vi "Main.vi"(11 "Module Admin":refnum<class "Delacor_lib_QMH_Module Admin.lvclass">) -> ()   [LabVIEW 2018, in "Application.lvlib"]
doc: "This template is based off of the Queued Message Handler design pattern and the Queued Message Handler project template that ships with LabVIEW.\n\nThe main difference is that the queue is private to this module and communication between modules is performed via Broadcast and Request events.\n\nRequest events are wrapped in public API methods and are handled in the Event Handling Loop (EHL) of this VI. Any module can register for Broadcast events sent by this module. The EHL generates messages based on user interface actions.\n\nThe Message Handling Loop (MHL) processes messages generated by the EHL, or by other messages. The messages are string values, so new messages can be added easily to the Message Cases case structure in the MHL. Each message cluster can also provide an optional value for Message Data, which is a variant that can be converted to whatever message-specific data is required.\n_____\nBased on DQMH Project Template 6.1.0.94."
uses:
  Application.lvlib
  <vilib>/Delacor/Delacor QMH/Libraries/Module Admin_class/Delacor_lib_QMH_Module Admin.lvclass
  Module Data--cluster.ctl
  <vilib>/Delacor/Delacor QMH/Libraries/Message Queue_class/Delacor_lib_QMH_Message Queue.lvclass/Delacor_lib_QMH_Message Queue.ctl
  Stop Argument--cluster.ctl
  <vilib>/Delacor/Delacor QMH/Libraries/Module Admin_class/Delacor_lib_QMH_Module Admin.lvclass/Delacor_lib_QMH_Module Admin.ctl
  <vilib>/Delacor/Delacor QMH/Libraries/Message Queue_class/Delacor_lib_QMH_Enqueue Message (Single).vi
  <vilib>/Delacor/Delacor QMH/Libraries/Module Admin_class/Delacor_lib_QMH_Get External Launch.vi
  <vilib>/Delacor/Delacor QMH/Libraries/Message Queue_class/Delacor_lib_QMH_Enqueue Message (Array).vi
  <vilib>/Utility/error.llb/Error Cluster From Error Code.vi
  <vilib>/ErrorRing/Error Ring.xnode
  <vilib>/Delacor/Delacor QMH/Libraries/Message Queue_class/Delacor_lib_QMH_Message Queue.lvclass
  Storage/Storage.lvlib
  DAQ/DAQ.lvlib
panel:
  in  "Virtual keyboard":bool
  out "设备状态":bool
  in  "Export Graph 3":bool
  in  "Export Graph 2":bool
  in  "通讯配置":bool
  in  "Clear Graph":bool
  in  "是否打开串口":bool
  in  "设备通讯":bool
  out "error out":errorcluster
  out "Status":string
  in  "Simulate MHL Error":bool
  in  "Simulate EHL Error":bool
  in  "Ring曲线选择":u16(ring) caption="选择查看曲线" items=["CH01", "CH02", "CH03", "CH04", "CH05", "CH06", "CH07", "CH08"]
  out "最高温度":dbl format="%#.0f℃"
  out "温度监控":T1 {"CH 8" format="%#0.1f℃"; "CH 7" format="%#0.1f℃"; "CH 6" format="%#0.1f℃"; "CH 5" format="%#0.1f℃"; "CH 4" format="%#0.1f℃"; "CH 3" format="%#0.1f℃"; "CH 2" format="%#0.1f℃"; "CH" format="%#0.1f℃"}
  out "Value":dbl caption="Y Value" format="%0.2f"
  out "XYGraph":cluster{"时间":dbl[], "曲线":dbl[]}(graph) caption="-- 温度曲线"
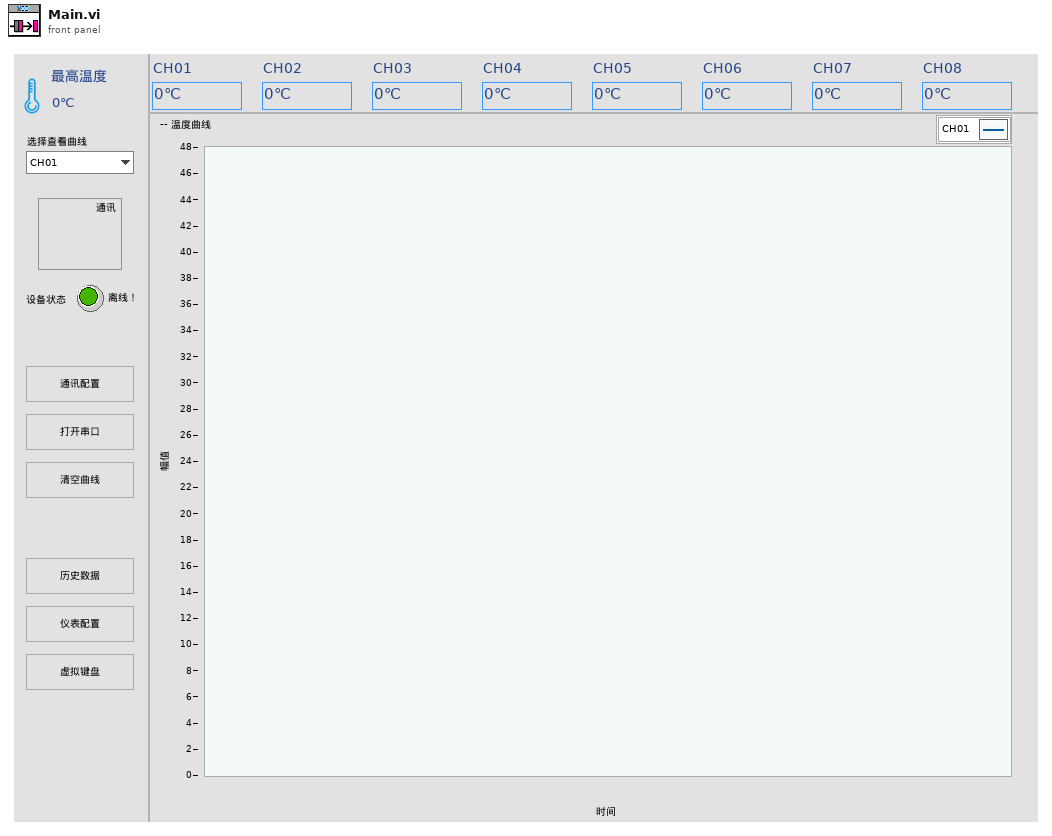
[diagram p1: front panel]
types:
  T1 = cluster{"CH":dbl, "CH 2":dbl, "CH 3":dbl, "CH 4":dbl, "CH 5":dbl, "CH 6":dbl, "CH 7":dbl, "CH 8":dbl}
  T2 = typedef "Storage.lvlib/Broadcast Events--cluster.ctl" = cluster{"Module Did Init":refnum<user-event>, "Status Updated":refnum<user-event>, "Error Reported":refnum<user-event>, "Module Did Stop":refnum<user-event>, "Update Module Execution Status":refnum<user-event>}
  T3 = typedef "DAQ.lvlib/Broadcast Events--cluster.ctl" = cluster{"Module Did Init":refnum<user-event>, "Status Updated":refnum<user-event>, "Error Reported":refnum<user-event>, "Module Did Stop":refnum<user-event>, "Update Module Execution Status":refnum<user-event>}
  T4 = typedef "Application.lvlib/Request Events--cluster.ctl" = cluster{"Stop Module":refnum<user-event>, "Show Panel":refnum<user-event>, "Hide Panel":refnum<user-event>, "Get Module Execution Status":refnum<user-event>, "Show Diagram":refnum<user-event>, "Wakeup or Sleep HL":refnum<user-event>}
  T5 = typedef "Application.lvlib/Module Data--cluster.ctl" = cluster{"Status":string, "TDMS":refnum<k34>}
  T6 = enum32{"invalid lock state", "Not Locked", "Locked (No Password)", "Password-protected"}
  T7 = typedef "Application.lvlib/Stop Argument--cluster.ctl" = cluster{"Origin":string, "Exit via Stop Module Req?":bool, "Wait for Module to stop?":bool}
  T8 = enum32{"Invalid", "Standard", "Closed", "Hidden", "Minimized", "Maximized"}
  T9 = typedef "LVPoint32TypeDef.ctl" = cluster{"Horizontal":i32, "Vertical":i32}
  T10 = cluster{"温度[0]":dbl, "温度[1]":dbl, "温度[2]":dbl, "温度[3]":dbl, "温度[4]":dbl, "温度[5]":dbl, "温度[6]":dbl, "温度[7]":dbl}
  T11 = typedef "LVPositionTypeDef.ctl" = cluster{"Left":i32, "Top":i32}
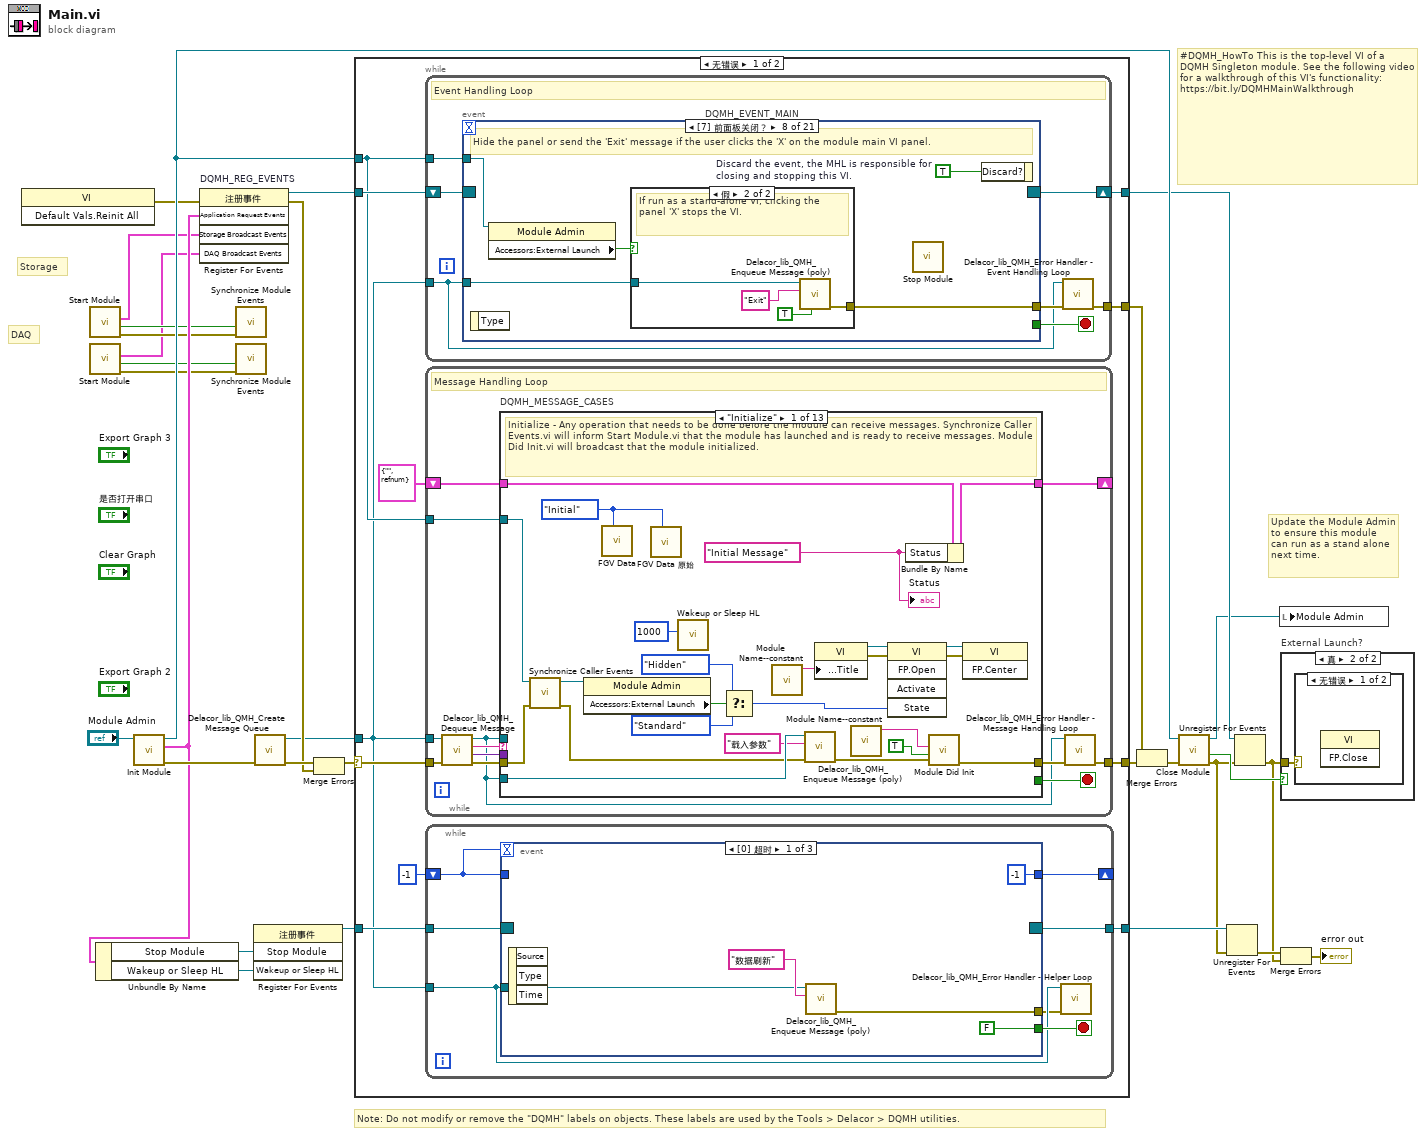
[diagram p0: block diagram]
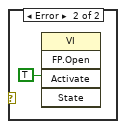
[diagram p3: hidden frame]
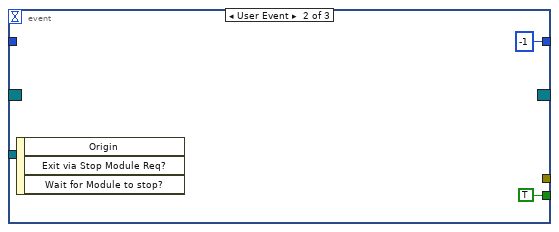
[diagram p4: hidden frame]
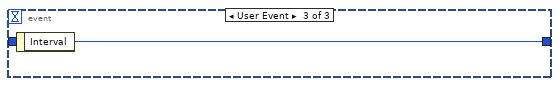
[diagram p5: hidden frame]
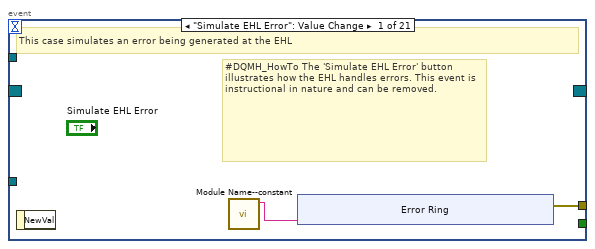
[diagram p6: hidden frame]
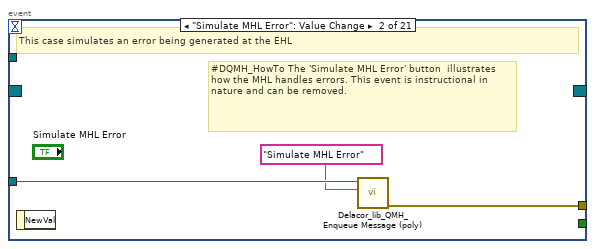
[diagram p7: hidden frame]
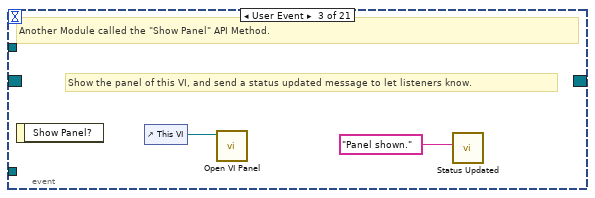
[diagram p8: hidden frame]
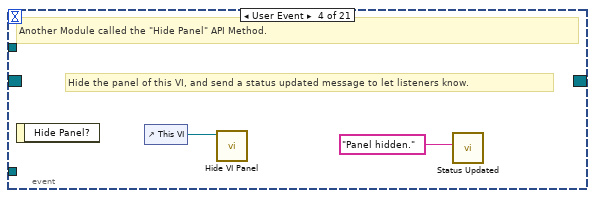
[diagram p9: hidden frame]
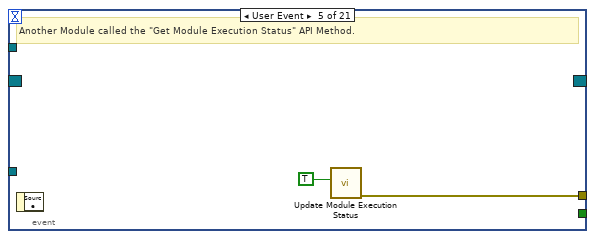
[diagram p10: hidden frame]
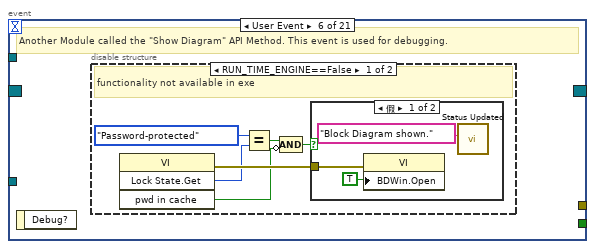
[diagram p11: hidden frame]
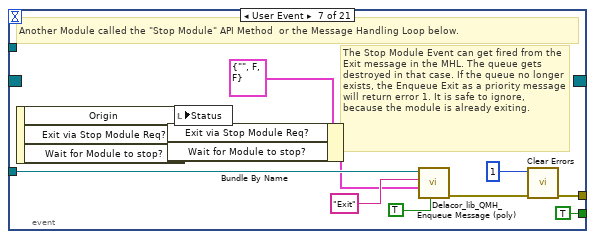
[diagram p14: hidden frame]
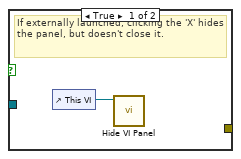
[diagram p15: hidden frame]
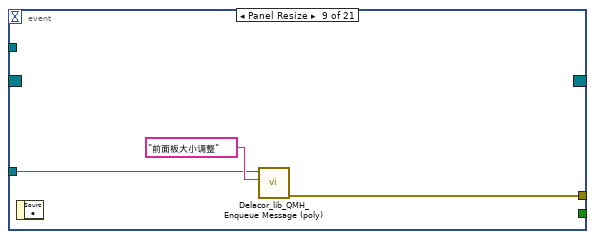
[diagram p16: hidden frame]
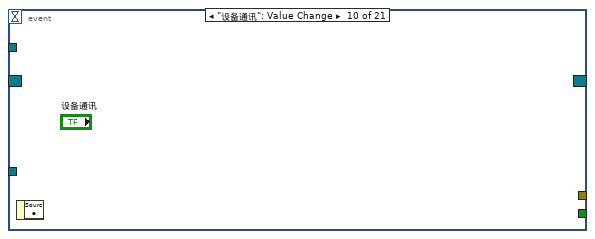
[diagram p17: hidden frame]
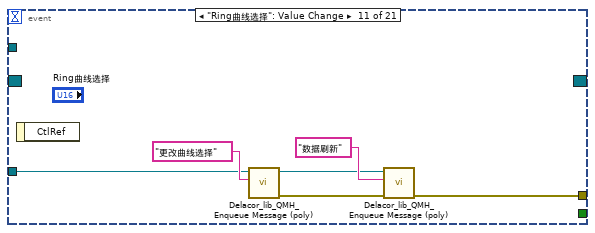
[diagram p18: hidden frame]
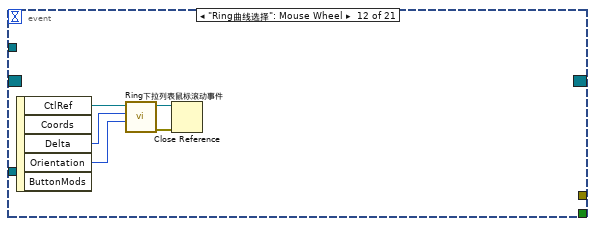
[diagram p19: hidden frame]
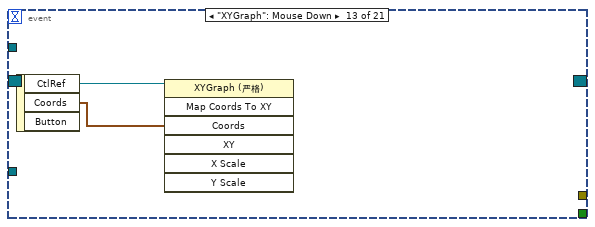
[diagram p20: hidden frame]
diagram:
  # "DAQ"
  # "Storage"
  # "#DQMH_HowTo This is the top-level VI of a DQMH Singleton module. See the following video for a walkthrough of this VI's functionality: https://bit.ly/DQMHMainWalkthrough"
  # "Note: Do not modify or remove the \"DQMH\" labels on objects. These labels are used by the Tools > Delacor > DQMH utilities."
  # "Update the Module Admin to ensure this module can run as a stand alone next time."
  n1 = invoke class="VI" method="Default Vals.Reinit All"() -> (error out=w7:errorcluster)  [unwired: 3 in, 2 out]
  n2 = call "Start Module.vi"() -> ("error out"=w4:errorcluster, "Wait for Event Sync?"=w6:bool, "Storage Broadcast Events"=w5:T2)  [unwired: 8 in, 1 out]
  n3 = call "Start Module.vi"() -> ("error out"=w1:errorcluster, "Wait for Event Sync?"=w3:bool, "DAQ Broadcast Events"=w2:T3)  [unwired: 8 in, 1 out]
  n4 = call "Init Module.vi"("Singleton Module Admin in"="Module Admin") -> ("error out"=w29:errorcluster, "Application Request Events"=w13:T4, "Singleton Module Admin out"=w23:refnum<class "Delacor_lib_QMH_Module Admin.lvclass">)  [unwired: 8 in]
  n5 = Unbundle By Name ("按名称解除捆绑")(w13) -> ("Stop Module"=w16:refnum<user-event>, "Wakeup or Sleep HL"=w15:refnum<user-event>)
  n6 = register-events "DQMH_REG_EVENTS"(error in=w7, w13, w5, w2) -> (reference out=w21:refnum<event-registration>, error out=w24:errorcluster)  [unwired: 1 in]
  n7 = call "Synchronize Module Events.vi"("error in"=w4, "Wait for Event Sync?"=w6) -> ()  [unwired: 9 in, 1 out]
  n8 = call "Synchronize Module Events.vi"("error in"=w1, "Wait for Event Sync?"=w3) -> ()  [unwired: 9 in, 1 out]
  n9 = register-events ("注册事件")(w16, w15) -> (reference out=w14:refnum<event-registration>)  [unwired: 2 in, 1 out]
  n10 = call <vilib>:"Delacor_lib_QMH_Create Message Queue.vi"("error in"=w29) -> ("error out"=w26:errorcluster, "Message Queue"=w20:refnum<class "Delacor_lib_QMH_Message Queue.lvclass">)  [unwired: 9 in]
  n11 = Merge Errors(w26, w24) -> (w25:errorcluster)
  n12 = case shown="无错误" w25 {
    selector: w25 -> [w39 w322]
    tunnel: [w41 w321] -> w30
    tunnel: [w38 w327] -> w22
    tunnel: w21 -> [w36 w327]
    tunnel: w20 -> [w32 w320]
    tunnel: [w40 _] -> w28
    tunnel: w23 -> [w35 w323]
    tunnel: w14 -> [w33 w319]
    tunnel: [w31 w319] -> w11
    frame No Error {
      n13 = while {
        tunnel: w32 -> [w57]
        shift-right: [w60] -> w38
        shift-left: w36 -> [w61]
        tunnel: [w62] -> w40
        tunnel: w35 -> [w58]
        stop <- w59 stop-if-true
        # "Event Handling Loop"
        n14 = event "DQMH_EVENT_MAIN" shown="[7] 前面板关闭？" {
          selector: w61 -> [_ _ _ _ _ _ _ _ _ _ _ _ _ _ _ _ _ _ _ _ _]
          dyn-events: [_ _ _ _ _ _ _ _ _ _ _ _ _ _ _ _ _ _ _ _ _] -> w60
          timeout: _ -> [_ _ _ _ _ _ _ _ _ _ _ _ _ _ _ _ _ _ _ _ _]
          tunnel: [_ _ _ _ _ _ TRUE ("Discard?") _ _ _ _ _ _ _ _ _ _ _ _ _ _] -> w59
          tunnel: w57 -> [_ w74 _ _ _ _ w98 w105 w114 _ w118 _ _ _ _ _ _ _ _ _ _]
          tunnel: [w65 w75 _ _ w81 _ w101 w107 w113 _ w120 _ _ _ _ _ _ _ _ _ _] -> w63
          tunnel: w58 -> [_ _ _ _ _ _ _ w104 _ _ _ _ _ _ _ _ _ _ _ _ _]
          event "Simulate EHL Error": Value Change {
            # "#DQMH_HowTo The 'Simulate EHL Error' button  illustrates how the EHL handles errors. This event is instructional in nature and can be removed."
            # "This case simulates an error being generated at the EHL"
            n15 = event-data() -> ()  [unwired: 1 in, 1 out]
            n16 = call "Module Name--constant.vi"() -> ("Module Name"=w64:string)  [unwired: 11 in]
            n17 = xnode "Error Ring"("参数 0"=w64) -> ("错误输出"=w65:errorcluster)
          }
          event "Simulate MHL Error": Value Change {
            # "#DQMH_HowTo The 'Simulate MHL Error' button  illustrates how the MHL handles errors. This event is instructional in nature and can be removed."
            # "This case simulates an error being generated at the EHL"
            n18 = event-data() -> ()  [unwired: 1 in, 1 out]
            n19 = call-poly <vilib>:"Delacor_lib_QMH_Enqueue Message (poly).vi"("Message"="Simulate MHL Error", "Message Queue in"=w74) -> ("error out"=w75:errorcluster)  [unwired: 8 in, 1 out]
          }
          event User Event {
            # "Show the panel of this VI, and send a status updated message to let listeners know."
            # "Another Module called the \"Show Panel\" API Method."
            n20 = event-data() -> ()  [unwired: 1 in, 1 out]
            n21 = control-ref of="This VI"() -> (w77:refnum<vi>)
            n22 = call "Open VI Panel.vi"("VI"=w77) -> ()  [unwired: 10 in, 1 out]
            n23 = call "Status Updated.vi"("Status"="Panel shown." ("format string")) -> ()  [unwired: 10 in, 1 out]
          }
          event User Event {
            # "Hide the panel of this VI, and send a status updated message to let listeners know."
            # "Another Module called the \"Hide Panel\" API Method."
            n24 = event-data() -> ()  [unwired: 1 in, 1 out]
            n25 = control-ref of="This VI"() -> (w79:refnum<vi>)
            n26 = call "Hide VI Panel.vi"("VI"=w79) -> ()  [unwired: 10 in, 1 out]
            n27 = call "Status Updated.vi"("Status"="Panel hidden." ("format string")) -> ()  [unwired: 10 in, 1 out]
          }
          event User Event {
            # "Another Module called the \"Get Module Execution Status\" API Method."
            n28 = event-data() -> ()  [unwired: 1 in, 1 out]
            n29 = call "Update Module Execution Status.vi"("Running?"=TRUE) -> ("error out"=w81:errorcluster)  [unwired: 10 in]
          }
          event User Event {
            # "Another Module called the \"Show Diagram\" API Method. This event is used for debugging."
            n30 = event-data() -> ()  [unwired: 1 in, 1 out]
            n31 = disable-structure shown="RUN_TIME_ENGINE==False" {
              frame condition #0 (active) {
                # "functionality not available in exe"
                n32 = invoke class="VI" method="Lock State.Get"() -> (error out=w87:errorcluster, "Get Lock State"=w86:T6, "pwd in cache"=w83:bool)  [unwired: 4 in, 1 out]
                n33 = Equal?(x=T6."Password-protected", y=w86) -> (x = y?=w84:bool)
                n34 = Compound Arithmetic op=AND(w84, invert w83) -> (w82:bool)
                n35 = case "条件结构" shown="假" w82 {
                  tunnel: w87 -> [w90 _]
                  frame False {
                    n36 = property class="VI"(error in=w90, "BDWin.Open"=TRUE ("Block Diagram Window:Open")) -> ()  [unwired: 1 in, 2 out]
                    n37 = call "Status Updated.vi"("Status"="Block Diagram shown." ("format string")) -> ()  [unwired: 10 in, 1 out]
                  }
                  frame True {
                    # "Password-protected VI, and the password is not in the cache. Do not show the diagram."
                  }
                }
              }
              frame condition #1 {
              }
            }
          }
          event User Event {
            # "The Stop Module Event can get fired from the Exit message in the MHL. The queue gets destroyed in that case. If the queue no longer exists, the Enqueue Exit as a priority message will return error 1. It is safe to ignore, because the module is already exiting."
            # "Another Module called the \"Stop Module\" API Method  or the Message Handling Loop below."
            n38 = event-data() -> ("Origin"=w97:string, "Exit via Stop Module Req?"=w93:bool, "Wait for Module to stop?"=w92:bool)  [unwired: 1 in]
            n39 = Bundle By Name(cluster=T7 {"Origin"="", "Exit via Stop Module Req?"=FALSE, "Wait for Module to stop?"=FALSE} ("Stop Argument"), "Exit via Stop Module Req?"=w93, "Wait for Module to stop?"=w92) -> (w91:T7)
            n40 = local write "Status"(w97) -> ()
            n41 = call-poly <vilib>:"Delacor_lib_QMH_Enqueue Message (poly).vi"("Priority Message? (F)"=TRUE, "Message Data"=w91, "Message"="Exit", "Message Queue in"=w98) -> ("error out"=w102:errorcluster)  [unwired: 6 in, 1 out]
            n42 = call <vilib>:"Clear Errors.vi"("error in (no error)"=w102, "specific error code to clear (0: all)"=1) -> ("error out"=w101:errorcluster)  [unwired: 4 in, 1 out]
          }
          event Panel Close? {
            w106 = TRUE  # Discard the event, the MHL is responsible for closing and stopping this VI.
            # "Hide the panel or send the 'Exit' message if the user clicks the 'X' on the module main VI panel."
            n43 = event-data() -> ()  [unwired: 1 in, 1 out]
            n44 = property class="Module Admin"(reference=w104) -> ("Accessors:External Launch"=w103:bool)  [unwired: 1 in, 2 out]
            n45 = case "条件结构" shown="假" w103 {
              tunnel: w105 -> [_ w111]
              tunnel: [_ w112] -> w107
              frame True {
                # "If externally launched, clicking the 'X' hides the panel, but doesn't close it."
                n46 = control-ref of="This VI"() -> (w108:refnum<vi>)
                n47 = call "Hide VI Panel.vi"("VI"=w108) -> ()  [unwired: 10 in, 1 out]
              }
              frame False {
                # "If run as a stand-alone VI, clicking the panel 'X' stops the VI."
                n48 = call-poly <vilib>:"Delacor_lib_QMH_Enqueue Message (poly).vi"("Priority Message? (F)"=TRUE, "Message"="Exit", "Message Queue in"=w111) -> ("error out"=w112:errorcluster)  [unwired: 7 in, 1 out]
              }
            }
            n49 = call "Stop Module.vi"() -> ()  [unwired: 11 in, 1 out]
            n50 = event-data("Discard?"=w106) -> ()  [unwired: 1 in, 1 out]
          }
          event Panel Resize {
            n51 = event-data() -> ()  [unwired: 1 in, 1 out]
            n52 = call-poly <vilib>:"Delacor_lib_QMH_Enqueue Message (poly).vi"("Message"="前面板大小调整", "Message Queue in"=w114) -> ("error out"=w113:errorcluster)  [unwired: 8 in, 1 out]
          }
          event "设备通讯": Value Change {
            n53 = event-data() -> ()  [unwired: 1 in, 1 out]
          }
          event "Ring曲线选择": Value Change {
            n54 = event-data() -> ()  [unwired: 1 in, 1 out]
            n55 = call-poly <vilib>:"Delacor_lib_QMH_Enqueue Message (poly).vi"("Message"="更改曲线选择", "Message Queue in"=w118) -> ("error out"=w116:errorcluster, "Message Queue out"=w117:refnum<class "Delacor_lib_QMH_Message Queue.lvclass">)  [unwired: 8 in]
            n56 = call-poly <vilib>:"Delacor_lib_QMH_Enqueue Message (poly).vi"("error in"=w116, "Message"="数据刷新", "Message Queue in"=w117) -> ("error out"=w120:errorcluster)  [unwired: 7 in, 1 out]
          }
          event "Ring曲线选择": Mouse Wheel {
            n57 = event-data() -> ("CtlRef"=w124:refnum<vi>, "Delta"=w122:i32, "Orientation"=w123:enum16{"Horizontal", "Vertical"})  [unwired: 1 in, 2 out]
            n58 = call "Ring下拉列表鼠标滚动事件.vi"("方向"=w123, "Delta"=w122, "CtlRef"=w124) -> ("error out"=w126:errorcluster, "CtlRef 2"=w125:refnum<vi>)  [unwired: 7 in]
            n59 = Close Reference(reference=w125, error in (no error)=w126) -> ()  [unwired: 1 out]
          }
          event "XYGraph": Mouse Down {
            n60 = event-data() -> ("CtlRef"=w128:refnum<vi>, "Coords"=w127:T9)  [unwired: 1 in, 1 out]
            n61 = invoke class="XYGraph (严格)" method="Map Coords To XY"(reference=w128, "Coords"=w127) -> ()  [unwired: 5 in, 7 out]
          }
          event "XYGraph": Mouse Down? {
            n62 = event-data() -> ("CtlRef"=w131:refnum<vi>, "Button"=w130:u16)  [unwired: 1 in, 2 out]
            n63 = case "条件结构" shown="1" w130 {
              tunnel: w131 -> [_ w136 w144]
              tunnel: [_ w132 w140] -> w129
              frame 0, Default {
              }
              frame 1 {
                n64 = property class="XYGraph (严格)"(reference=w136) -> (reference out=w134:refnum<vi>, "ActPaletteTool"=w135:i32)  [unwired: 1 in, 1 out]
                n65 = Equal To 0?(x=w135) -> (x = 0?=w133:bool)
                n66 = Not(x=w133) -> (.not. x?=w132:bool)
                n67 = case "条件结构" shown="假" w133 {
                  tunnel: w134 -> [w138 _]
                  frame False {
                    n68 = property class="XYGraph (严格)"(reference=w138, "ActPaletteTool"=0 ("选板:活动工具")) -> ()  [unwired: 1 in, 2 out]
                  }
                  frame True {
                  }
                }
              }
              frame 3 {
                n69 = property class="XYGraph (严格)"(reference=w144) -> (reference out=w142:refnum<vi>, "ActPaletteTool"=w143:i32)  [unwired: 1 in, 1 out]
                n70 = Equal?(x=1, y=w143) -> (x = y?=w141:bool)
                n71 = Not(x=w141) -> (.not. x?=w140:bool)
                n72 = case "条件结构" shown="假" w141 {
                  tunnel: w142 -> [w146 _]
                  frame False {
                    n73 = property class="XYGraph (严格)"(reference=w146, "ActPaletteTool"=1 ("选板:活动工具")) -> ()  [unwired: 1 in, 2 out]
                  }
                  frame True {
                  }
                }
              }
            }
            n74 = event-data("Discard?"=w129) -> ()  [unwired: 1 in, 1 out]
          }
          event "XYGraph": Mouse Enter {
            w147 = TRUE ("游标.可见")
            n75 = event-data() -> ("CtlRef"=w148:refnum<vi>)  [unwired: 1 in]
            n76 = property class="XYGraph (严格)"(reference=w148, "Cursor.Visible"=w147) -> (reference out=w149:refnum<vi>)  [unwired: 1 in, 1 out]
            n77 = property on="Value" class="DigNum (严格)"("Visible"=w147) -> ()  [unwired: 2 in, 2 out]
            n78 = Close Reference(reference=w149) -> ()  [unwired: 1 in, 1 out]
          }
          event "XYGraph": Mouse Leave {
            w151 = FALSE ("游标.可见")
            n79 = event-data() -> ("CtlRef"=w152:refnum<vi>)  [unwired: 1 in]
            n80 = property class="XYGraph (严格)"(reference=w152, "Cursor.Visible"=w151) -> (reference out=w153:refnum<vi>)  [unwired: 1 in, 1 out]
            n81 = property on="Value" class="DigNum (严格)"("Visible"=w151, "Value"=0.0) -> ()  [unwired: 2 in, 2 out]
            n82 = Close Reference(reference=w153) -> ()  [unwired: 1 in, 1 out]
          }
          event "XYGraph": Mouse Move {
            n83 = event-data() -> ("CtlRef"=w159:refnum<vi>, "Coords"=w158:T9)  [unwired: 1 in]
            n84 = invoke class="XYGraph (严格)" method="Map Coords To XY"(reference=w159, "Coords"=w158) -> (reference out=w157:refnum<vi>, "XY"=w155:cluster{"X":dbl, "Y":dbl})  [unwired: 5 in, 5 out]
            n85 = property class="XYGraph (严格)"(reference=w157, "Cursor.Cursor Position"=w155, "Cursor.Visible"=TRUE ("游标.可见")) -> ()  [unwired: 1 in, 2 out]
            n86 = Unbundle(w155) -> ("Y"=→"Value":dbl)  [unwired: 1 out]
          }
          event "Clear Graph": Mouse Up {
            n87 = event-data() -> ()  [unwired: 1 in, 8 out]
          }
          event "Clear Graph": Mouse Wheel {
            n88 = event-data() -> ()  [unwired: 1 in, 8 out]
          }
          event "通讯配置": Value Change {
            n89 = event-data() -> ("CtlRef"=w160:refnum<vi>)  [unwired: 1 in, 5 out]
            n90 = invoke class="Bool (严格)" method="Reinit To Default"(reference=w160) -> ()  [unwired: 2 in, 3 out]
            n91 = call "Form_设备通讯配置 Start Module.vi"() -> ("error out"=w161:errorcluster, "VI引用句柄"=w162:refnum<vi>)  [unwired: 10 in]
            n92 = Close Reference(reference=w162, error in (no error)=w161) -> ()  [unwired: 1 out]
          }
          event "Virtual keyboard": Value Change {
            n93 = event-data() -> ("CtlRef"=w163:refnum<vi>)  [unwired: 1 in, 5 out]
            n94 = invoke class="Bool (严格)" method="Reinit To Default"(reference=w163) -> ()  [unwired: 2 in, 3 out]
            n95 = call "Windows虚拟键盘调用.vi"() -> ()  [unwired: 11 in, 1 out]
          }
        }
        n96 = call-dynamic "Delacor_lib_QMH_Error Handler - Event Handling Loop.vi"("error in"=w63, "Message Queue in"=w57) -> ("dup error in"=w62:errorcluster)  [unwired: 8 in, 1 out]
      }
      n97 = while {
        tunnel: w32 -> [w166]
        shift-right: [w170] -> _
        shift-left: T5 {"Status"="", "TDMS"=refnum} ("Data Cluster") -> [w171]
        tunnel: w39 -> [w174]
        tunnel: [w172] -> w41
        tunnel: w35 -> [w165]
        stop <- w169 stop-if-true
        # "Message Handling Loop"
        n98 = call-dynamic "Delacor_lib_QMH_Dequeue Message.vi"("error in"=w174, "Message Queue in"=w166) -> ("error out"=w173:errorcluster, "Message Data"=w167:variant, "Message"=w168:string, "Message Queue out"=w164:refnum<class "Delacor_lib_QMH_Message Queue.lvclass">)  [unwired: 6 in]
        n99 = case "DQMH_MESSAGE_CASES" shown="\"Initialize\"" w168 {
          selector: w168 -> [_ _ _ _ _ _ _ _ _ _ _ _ w306]
          tunnel: w164 -> [_ _ _ _ w224 _ _ _ _ _ w276 w298 _]
          tunnel: w173 -> [w197 w206 w212 w215 w223 w236 w252 w259 w261 w266 w283 w304 w308]
          tunnel: [w196 w206 w212 w214 w222 w236 w252 w259 w261 w265 w279 w301 w309] -> w175
          tunnel: w171 -> [w187 w205 w211 w213 w220 w235 w251 w258 w260 w263 w278 w297 w307]
          tunnel: [w186 w205 w211 w213 w218 w235 w251 w258 w260 w263 w278 w297 w307] -> w170
          tunnel: [_ _ _ _ _ _ _ _ _ _ _ w296 _] -> w169
          tunnel: w167 -> [_ _ _ _ _ _ _ _ _ _ w277 w295 _]
          tunnel: w165 -> [w188 _ _ _ _ _ _ _ _ _ w275 w290 _]
          tunnel: w164 -> [w180 _ _ _ _ _ _ _ _ _ _ _ _]
          frame "Initialize" {
            w176 = enum16{"Initial", "Read", "Write"}."Initial" ("Action")
            w182 = "Initial Message" ("Initial Message")
            # "Initialize - Any operation that needs to be done before the module can receive messages. Synchronize Caller Events.vi will inform Start Module.vi that the module has launched and is ready to receive messages. Module Did Init.vi will broadcast that the module initialized."
            n100 = call "Synchronize Caller Events.vi"("error in (no error)"=w197, "Singleton Module Admin in"=w188) -> ("error out"=w179:errorcluster, "Singleton Module Admin out"=w183:refnum<class "Delacor_lib_QMH_Module Admin.lvclass">)  [unwired: 8 in]
            n101 = property class="Module Admin"(reference=w183) -> ("Accessors:External Launch"=w192:bool)  [unwired: 1 in, 2 out]
            n102 = call "FGV Data.vi"("Action"=w176) -> ()  [unwired: 9 in, 2 out]
            n103 = call "FGV Data 原始.vi"("Action"=w176) -> ()  [unwired: 9 in, 2 out]
            n104 = call "Wakeup or Sleep HL.vi"("Interval"=1000) -> ()  [unwired: 10 in, 1 out]
            n105 = Select(t=T8."Hidden" ("State"), s=w192, f=T8."Standard" ("State")) -> (s? t:f=w189:T8)
            n106 = call "Module Name--constant.vi"() -> ("Module Name"=w195:string)  [unwired: 11 in]
            n107 = call-poly <vilib>:"Delacor_lib_QMH_Enqueue Message (poly).vi"("error in"=w179, "Message"="载入参数", "Message Queue in"=w180) -> ("error out"=w178:errorcluster)  [unwired: 7 in, 1 out]
            n108 = property class="VI"("Front Panel.Title"=w195) -> (reference out=w194:refnum<vi>, error out=w199:errorcluster)  [unwired: 2 in]
            n109 = call "Module Name--constant.vi"() -> ("Module Name"=w184:string)  [unwired: 11 in]
            n110 = invoke class="VI" method="FP.Open"(reference=w194, error in=w199, "State"=w189) -> (reference out=w193:refnum<vi>, error out=w198:errorcluster)  [unwired: 2 in, 3 out]
            n111 = Bundle By Name(cluster=w187, "Status"=w182) -> (w186:T5)
            n112 = call "Module Did Init.vi"("error in (no error)"=w178, "Initialized?"=TRUE, "Origin"=w184) -> ("error out"=w196:errorcluster)  [unwired: 8 in]
            n113 = invoke class="VI" method="FP.Center"(reference=w193, error in=w198) -> ()  [unwired: 1 in, 3 out]
            "Status" <- w182
          }
          frame "载入参数" {
            w200 = u32 11776947 ("颜色盒")
            n114 = Bundle("颜色盒"=w200, "颜色盒"=w200) -> (w201:cluster{"颜色盒":u32, "颜色盒":u32})  [unwired: 1 in]
            n115 = property on="分隔栏" class="Splitter"("Colors"=w201) -> ()  [unwired: 2 in, 2 out]
            n116 = property on="分隔栏 2" class="Splitter"("Colors"=w201) -> ()  [unwired: 2 in, 2 out]
            n117 = control-ref of="Ring曲线选择"() -> (w203:refnum<vi>)
            n118 = for {
              N: 8 -> [_]
              tunnel: [w207] -> w204 mode=indexing
              i -> [w210]
              n119 = Increment(x=w210) -> (x+1=w209:i32)
              n120 = Format Into String(format string="CH0%d" ("格式字符串"), w209) -> (resulting string=w207:string)  [unwired: 2 in, 1 out]
            }
            n121 = property class="Ring (严格)"(reference=w203, "Strings []"=w204) -> ()  [unwired: 1 in, 2 out]
          }
          frame "---Module Specific---" {
            # "Separator -- The following cases handle messages specific to this Module."
          }
          frame "---Copy This Frame---" {
            # "Duplicate this frame when creating new messages.  Change this comment in the duplicated frame to describe this message."
            n122 = Merge Errors(w215) -> (w214:errorcluster)
          }
          frame "数据刷新" {
            n123 = Unbundle By Name(w220) -> ("TDMS"=w216:refnum<k34>)
            n124 = Not A Number/Path/Refnum?(number/path/refnum=w216) -> (NaN/Path/Refnum?=w219:bool)
            n125 = case shown="真" w219 {
              tunnel: [w226 w227] -> w217
              tunnel: w216 -> [w226 _]
              frame False {
              }
              frame True {
                n126 = call "Get TDMS Ref.vi"("TDMS ID"=0) -> ("TDMS"=w227:refnum<k34>)  [unwired: 8 in, 2 out]
              }
            }
            n127 = call-poly <vilib>:"Delacor_lib_QMH_Enqueue Message (poly).vi"("error in"=w223, "Message Array"=string[] ["刷新曲线"] ("Message"), "Message Queue in"=w224) -> ("error out"=w222:errorcluster)  [unwired: 7 in, 1 out]
            n128 = Bundle By Name(cluster=w220, "TDMS"=w217) -> (w218:T5)
            n129 = call "Wakeup or Sleep HL.vi"("Interval"=1000) -> ()  [unwired: 10 in, 1 out]
          }
          frame "刷新曲线" {
            n130 = Unbundle By Name(w235) -> ("TDMS"=w233:refnum<k34>)
            n131 = call "FGV Data.vi"("Action"=enum16{"Initial", "Read", "Write"}."Read") -> ("Data OUT"=w231:cluster{"Con?":bool, "温度":dbl[]})  [unwired: 9 in, 1 out]
            n132 = Unbundle By Name(w231) -> ("Con?"=→"设备状态":bool, "温度"=w230:dbl[])
            n133 = Not A Number/Path/Refnum?(number/path/refnum=w233) -> (NaN/Path/Refnum?=w234:bool)
            n134 = case shown="假" w234 {
              tunnel: w233 -> [w243 _]
              tunnel: w230 -> [w237 _]
              frame False {
                n135 = property on="Ring曲线选择" class="Ring (严格)"() -> ("RingText.Text"=w240:string)  [unwired: 2 in, 2 out]
                n136 = Array To Cluster(array=w237) -> (cluster=→"温度监控":T10)
                n137 = Array Max & Min(array=w237) -> (max value=→"最高温度":dbl)  [unwired: 3 out]
                n138 = call "TDMS_数据读取.vi"("总数（-1:全部）"=i64 300, "CH Name[]"=w240, "组名称"="温度", "tdms文件"=w243) -> ("error out"=w242:errorcluster, "曲线"=→"XYGraph":cluster{"时间":dbl[], "曲线":dbl[]})  [unwired: 3 in, 3 out]
                n139 = call <vilib>:"Clear Errors.vi"("error in (no error)"=w242) -> ()  [unwired: 5 in, 2 out]
              }
              frame True {
              }
            }
          }
          frame "前面板大小调整" {
            n140 = control-ref of="本VI"() -> (w250:refnum<vi>)
            n141 = control-ref of="温度监控"() -> (w249:refnum<vi>)
            n142 = call "数值簇元素排列适应窗格.vi"("引用"=w250) -> ()  [unwired: 10 in, 1 out]
            n143 = property on="属性节点" class="Clust (严格)" props=["Height", "Width"](reference=w249) -> ("Height"=w247:u32)  [unwired: 1 in, 3 out]
            n144 = property on="分隔栏 2" class="Splitter"() -> (error out=w248:errorcluster, "Position"=w246:T11)  [unwired: 2 in, 1 out]
            n145 = property on="分隔栏 2" class="Splitter"(error in=w248, "Position"=w247, "Position"=w246) -> ()  [unwired: 1 in, 2 out]
            n146 = property on="Value" class="DigNum (严格)"("Position"=w246) -> ()  [unwired: 2 in, 2 out]
          }
          frame "更改曲线选择" {
            n147 = control-ref of="Ring曲线选择"() -> (w254:refnum<vi>)
            n148 = control-ref of="XYGraph"() -> (w255:refnum<vi>)
            n149 = property class="Ring (严格)"(reference=w254) -> ("RingText.Text"=w253:string)  [unwired: 1 in, 2 out]
            n150 = property on="属性节点" class="XYGraph (严格)"(reference=w255, "Active Plot"=u32 0 ("活动曲线"), "LegNumRows"=u32 1 ("图例:行数"), "Plot.Plot Name"=w253) -> ()  [unwired: 1 in, 2 out]
          }
          frame "---Exit and Error Handling---" {
            # "Separator - The following cases handle errors and exit messages."
          }
          frame "Simulate MHL Error" {
            # "#DQMH_HowTo The 'Simulate MHL Error' button  illustrates how the MHL handles errors. This event is instructional in nature and can be removed."
            # "Simulate an error occurring at the MHL"
            n151 = call "Module Name--constant.vi"() -> ("Module Name"=w262:string)  [unwired: 11 in]
            n152 = xnode "Error Ring"("参数 0"=w262) -> ("错误输出"=w264:errorcluster)
            n153 = Merge Errors(w266, w264) -> (w265:errorcluster)
          }
          frame "Error" {
            # "#CodeRecommended - If you ever change the name of this \"Error\" message, you'll need to update the name in the Check Loop Error.vi as well."
            # "#CodeRecommended - If the module is running in standalone mode (External Launch = FALSE), this code will pop up an error dialog and call the 'Exit' message if an error occurs. Add more fine-grained error handling here."
            # "Error - Check the error message data and respond accordingly. This message is sent by the \"Error Handler\" VIs at the end of each loop in this application."
            n154 = property class="Module Admin"(reference=w275) -> ("Accessors:External Launch"=w274:bool)  [unwired: 1 in, 2 out]
            n155 = Variant To Data(error in=w283, type=errorcluster {"status"=FALSE, "code"=0, "source"=""} ("error constant"), Variant=w277) -> (data=w284:errorcluster, error out=w281:errorcluster)
            n156 = call "Error Reported.vi"("Error"=w284) -> ()  [unwired: 10 in, 1 out]
            n157 = case shown="假" w274 {
              tunnel: [w289 _] -> w280
              tunnel: w276 -> [w287 _]
              tunnel: w284 -> [w288 _]
              frame False {
                # "If the module is running standalone, then pop up an error dialog and call the \"Exit\" message."
                n158 = call <vilib>:"Simple Error Handler.vi"("error in (no error)"=w288) -> ()  [unwired: 4 in, 5 out]
                n159 = call-poly <vilib>:"Delacor_lib_QMH_Enqueue Message (poly).vi"("Priority Message? (F)"=TRUE, "Message"="Exit", "Message Queue in"=w287) -> ("error out"=w289:errorcluster)  [unwired: 7 in, 1 out]
              }
              frame True {
                # "If the module was launched externally, calling the Error Reported broadcast VI is the only action performed by the \"Error\" message. The module's caller can then process the error appropriately."
              }
            }
            n160 = Merge Errors(w281, w280) -> (w279:errorcluster)
            n161 = local write "error out"(w279) -> ()
          }
          frame "Exit" {
            w294 = 91  # 91: not all Exit messages will have an argument
            w296 = TRUE  # Stop the VI
            # "DAQ"
            # "Storage"
            # "Release the message queue reference"
            # "#CodeNeeded - Add any required cleanup code here"
            # "Exit - Exit the application."
            n162 = Variant To Data(error in=w304, type=T7 {"Origin"="", "Exit via Stop Module Req?"=FALSE, "Wait for Module to stop?"=FALSE} ("Stop Argument"), Variant=w295) -> (data=w292:T7, error out=w300:errorcluster)
            n163 = call <vilib>:"Clear Errors.vi"("error in (no error)"=w300, "specific error code to clear (0: all)"=w294) -> ("error out"=w303:errorcluster)  [unwired: 4 in, 1 out]
            n164 = control-ref of="This VI"() -> (w291:refnum<vi>)
            n165 = call-dynamic "Delacor_lib_QMH_Release Message Queue.vi"("error in"=w303, "Message Queue"=w298) -> ("error out"=w302:errorcluster)  [unwired: 9 in]
            n166 = call "Handle Exit.vi"("Stop Argument"=w292, "Admin in"=w290, "VI reference"=w291) -> ("error out"=w299:errorcluster)  [unwired: 7 in, 1 out]
            n167 = Merge Errors(w302, w299) -> (w301:errorcluster)
            n168 = call "Stop Module.vi"() -> ()  [unwired: 11 in, 1 out]
            n169 = call "Stop Module.vi"() -> ()  [unwired: 11 in, 1 out]
          }
          frame Default {
            # "'Default' case only runs if there is a message that isn't defined in any of the other cases.  Output a programming error."
            n170 = call "Module Name--constant.vi"() -> ("Module Name"=w305:string)  [unwired: 11 in]
            n171 = xnode "Error Ring"("参数 0"=w306, "参数 1"=w305) -> ("错误输出"=w310:errorcluster)
            n172 = Merge Errors(w308, w310) -> (w309:errorcluster)
          }
        }
        n173 = call-dynamic "Delacor_lib_QMH_Error Handler - Message Handling Loop.vi"("error in"=w175, "Message Queue in"=w164) -> ("dup error in"=w172:errorcluster)  [unwired: 8 in, 1 out]
      }
      n174 = while {
        shift-right: [w47] -> _
        shift-left: -1 ("Interval") -> [w48]
        tunnel: w33 -> [w45]
        tunnel: [w44] -> w31
        tunnel: w32 -> [w43]
        stop <- w46 stop-if-true
        n175 = event "事件结构" shown="[0] 超时" {
          selector: w45 -> [_ _ _]
          dyn-events: [_ _ _] -> w44
          timeout: w48 -> [_ _ _]
          tunnel: w48 -> [_ _ _]
          tunnel: [-1 ("Interval") -1 w56] -> w47
          tunnel: [FALSE TRUE _] -> w46
          tunnel: w43 -> [w51 _ _]
          tunnel: [w50 _ _] -> w42
          event Timeout {
            n176 = event-data() -> ()  [unwired: 1 in, 3 out]
            n177 = call-poly <vilib>:"Delacor_lib_QMH_Enqueue Message (poly).vi"("Message"="数据刷新", "Message Queue in"=w51) -> ("error out"=w50:errorcluster)  [unwired: 8 in, 1 out]
          }
          event User Event {
            n178 = event-data() -> ()  [unwired: 1 in, 3 out]
          }
          event User Event {
            n179 = event-data() -> ("Interval"=w56:i32)  [unwired: 1 in]
          }
        }
        n180 = call-dynamic "Delacor_lib_QMH_Error Handler - Helper Loop.vi"("error in"=w42, "Message Queue in"=w43) -> ()  [unwired: 8 in, 2 out]
      }
    }
    frame Error {
      # "Synchronize Caller Events.vi will inform Start Module.vi that the module has launched and will let the code calling Start Module.vi register for broadcasts and would permit the caller receive the broadcast that an error occurred at launch time."
      n181 = call-dynamic "Delacor_lib_QMH_Release Message Queue.vi"("error in"=w322, "Message Queue"=w320) -> ("error out"=w321:errorcluster)  [unwired: 9 in]
      n182 = call "Synchronize Caller Events.vi"("Singleton Module Admin in"=w323) -> ("error out"=w328:errorcluster)  [unwired: 9 in, 1 out]
      n183 = call "Module Name--constant.vi"() -> ("Module Name"=w326:string)  [unwired: 11 in]
      n184 = Format Into String(format string="An error occurred during initialization. %s is no longer running.", w326) -> (resulting string=w324:string)  [unwired: 2 in, 1 out]
      n185 = Merge Errors(w321, w328) -> (w329:errorcluster)
      n186 = call "Error Reported.vi"("Additional Information"=w324, "Error"=w329) -> ()  [unwired: 9 in, 1 out]
    }
  }
  n187 = Merge Errors(w28, w30) -> (w27:errorcluster)
  n188 = call "Close Module.vi"("error in (no error)"=w27, "Module Admin in"=w23) -> ("error out"=w10:errorcluster, "External Launch"=w17:bool, "Module Admin out"=w18:refnum<class "Delacor_lib_QMH_Module Admin.lvclass">)  [unwired: 7 in]
  n189 = Unregister For Events(event registration refnum=w11, error in=w10) -> (error out=w12:errorcluster)
  n190 = Unregister For Events(event registration refnum=w22, error in=w10) -> (error out=w9:errorcluster)
  n191 = local write "Module Admin"(w18) -> ()
  n192 = case "External Launch?" shown="真" w17 {
    tunnel: w9 -> [_ w330]
    frame False {
    }
    frame True {
      n193 = case "条件结构" shown="无错误" w330 {
        frame No Error {
          n194 = invoke class="VI" method="FP.Close"() -> ()  [unwired: 3 in, 3 out]
        }
        frame Error {
          n195 = invoke class="VI" method="FP.Open"("Activate"=TRUE ("Activate?")) -> ()  [unwired: 4 in, 5 out]
        }
      }
    }
  }
  n196 = Merge Errors(w12, w9) -> (→"error out":errorcluster)
